vi "Set Matrix - file.vi"(5 "double array":dbl[][](array[numeric]), 6 "cmplx double array":cdb[][](array[numeric]), 7 "string array":string[](array[string]), 8 "error in (no error)":errorcluster, 10 "variable name":string, 11 "GOLPI ref. in":T1={"pipe handle"={"lv_proc.dll file path"=path "", "process instance handle"=[], "debug mode"=FALSE, "debug data"=[]}, "fast read timeout [ms]"=500, "fast read settle time [ms]"=10, "fast read to multiple [ms]"=1, "max elements per input line"=100, "slow read timeout [ms]"=5000, "stdin double format specifier"="%_16e", "max elements per stdout output column"=100, "console mode bitstream"=FALSE, "bitstream first read timeout [ms]"=1000, "bitstream read timeout [ms]"=50, "struct transfer possible"=FALSE}) -> (0 "error out":errorcluster, 3 "GOLPI ref. out":T1={"pipe handle"={"lv_proc.dll file path"=path "", "process instance handle"=[], "debug mode"=FALSE, "debug data"=[]}, "fast read timeout [ms]"=500, "fast read settle time [ms]"=10, "fast read to multiple [ms]"=1, "max elements per input line"=100, "slow read timeout [ms]"=5000, "stdin double format specifier"="%_16e", "max elements per stdout output column"=100, "console mode bitstream"=FALSE, "bitstream first read timeout [ms]"=1000, "bitstream read timeout [ms]"=50, "struct transfer possible"=FALSE})   [LabVIEW 2013, in "GOLPI library.lvlib"]
doc: "Saves LabVIEW variable into temporary file and loads it into GNU Octave. Supported are reals (doubles), complex and strings. Only one input can be nonempty array."
uses:
  GOLPI library.lvlib
  Public/GOLPI reference Type Def.ctl
  LV Process source distribution/Pipe Handle.ctl
  Type Definitions/Custom Error Codes Enum Type Def.vi
  LV Process source distribution/LV Process library.lvlib
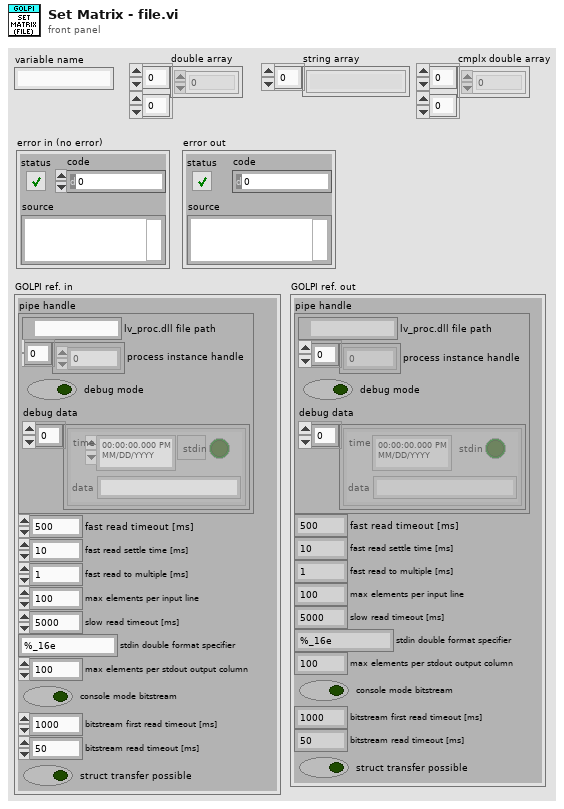
[diagram p1: front panel]
types:
  T1 = typedef "GOLPI library.lvlib/GOLPI reference Type Def.ctl" = cluster{"pipe handle":T2, "fast read timeout [ms]":u32, "fast read settle time [ms]":u32, "fast read to multiple [ms]":u32, "max elements per input line":u32, "slow read timeout [ms]":u32, "stdin double format specifier":string, "max elements per stdout output column":u32, "console mode bitstream":bool, "bitstream first read timeout [ms]":u32, "bitstream read timeout [ms]":u32, "struct transfer possible":bool}
  T2 = typedef "LV Process library.lvlib/Pipe Handle.ctl" = cluster{"lv_proc.dll file path":path, "process instance handle":u32[], "debug mode":bool, "debug data":cluster{"time":timestamp, "stdin":bool, "data":string}[]}
  T3 = typedef "GOLPI library.lvlib/Custom Error Codes Enum Type Def.vi" = enum16{"no error", "00 working directory PAR1 missing", "01 octave binary PAR1 missing", "02 octave report error PAR1", "03 empty output last cmd PAR1", "04 missing temporary file PAR1", "05 pwd PAR 1 not exist", "06 oct package not installed", "10 var PAR1 not string, vect", "11 var PAR1 not num, scal, ~compl", "12 var PAR1 not num, scal, compl", "13 var PAR1 not num, vect, ~compl", "14 var PAR1 not num, vect, compl", "15 var PAR1 not num, mat, ~compl", "16 var PAR1 not num, mat, ~compl", "30 read timeout", "60 bitstream transport failed", "61 bitstream decode error PAR1", "62 bitstream cannot be set", "70 struct transfer not possible", "80 struct: cluster elem. PAR1 not implem.", "81 struct: structure field PAR1 not implem.", "82 struct: size mismatch of PAR1", "83 struct: type mismatch of PAR1", "98 internal error", "99 not finished"}
  T4 = enum16{"open", "replace", "create", "open or create", "replace or create", "replace or create with confirmation"}
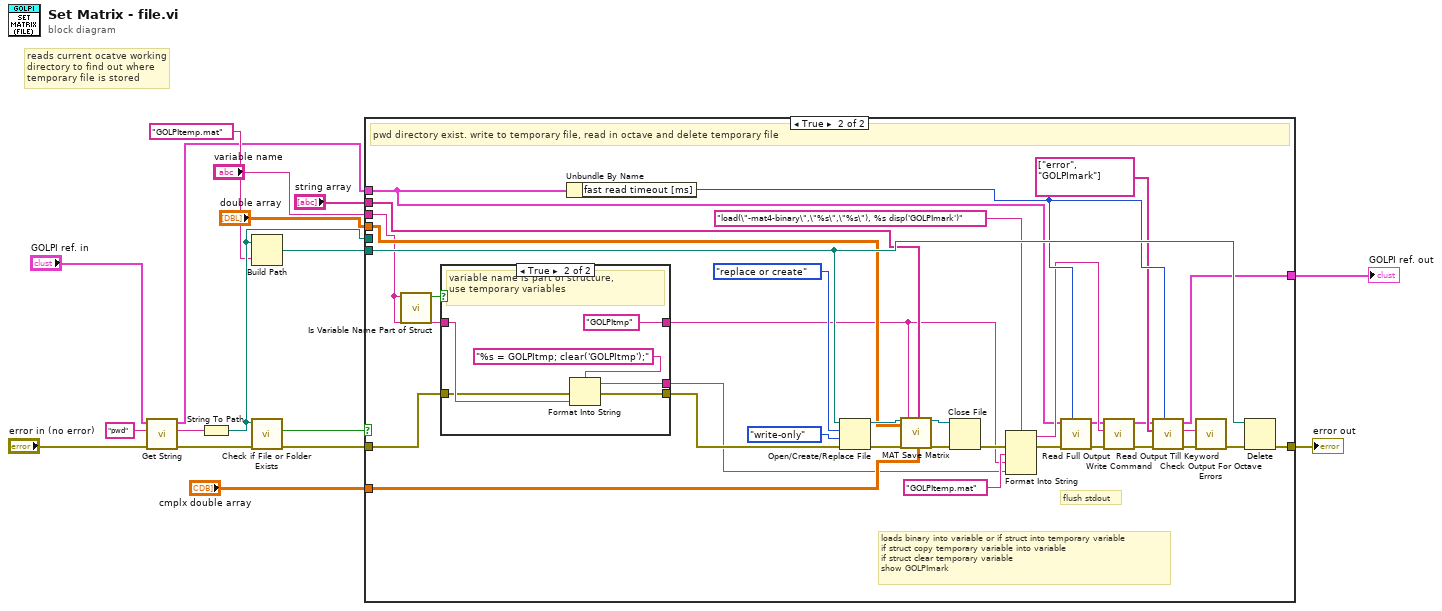
[diagram p0: block diagram]
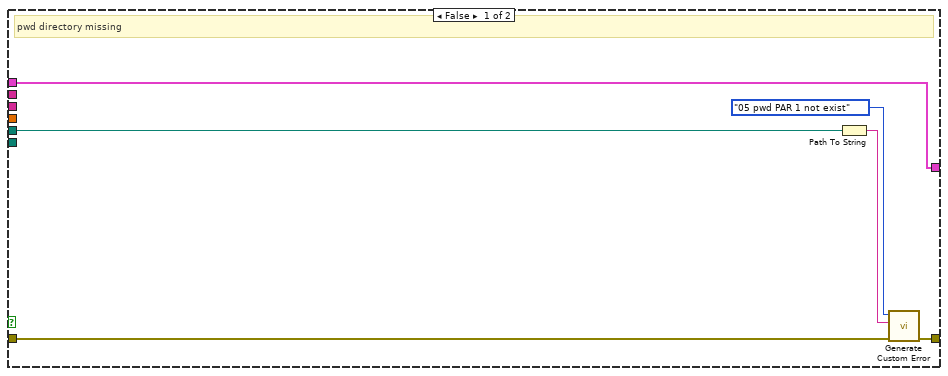
[diagram p2: hidden frame]
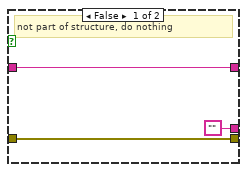
[diagram p3: hidden frame]
diagram:
  # "reads current ocatve working\ndirectory to find out where\ntemporary file is stored"
  n1 = call "Get String.vi"("error in"="error in (no error)", "variable name"="pwd", "GOLPI ref. in"="GOLPI ref. in") -> ("error out"=w7:errorcluster, "value"=w5:string, "GOLPI ref. out"=w1:T1)  [unwired: 6 in]
  n2 = String To Path(string=w5) -> (path=w3:path)
  n3 = Build Path(base path=w3, name or relative path="GOLPItemp.mat") -> (appended path=w4:path)
  n4 = call <vilib>:"Check if File or Folder Exists.vi"("error in (no error)"=w7, "path"=w3) -> ("error out"=w9:errorcluster, "file or folder exists?"=w8:bool)  [unwired: 7 in, 1 out]
  n5 = case shown="True" w8 {
    tunnel: [w22 w54] -> w17
    tunnel: w9 -> [w23 w27]
    tunnel: w4 -> [_ w53]
    tunnel: w3 -> [w19 _]
    tunnel: "variable name" -> [_ w28]
    tunnel: "string array" -> [_ w48]
    tunnel: "double array" -> [_ w47]
    tunnel: "cmplx double array" -> [_ w46]
    tunnel: w1 -> [w18 w31]
    tunnel: [w18 w30] -> w10
    frame False {
      # "pwd directory missing"
      n6 = Path To String(path=w19) -> (string=w20:string)
      n7 = call "Generate Custom Error.vi"("error in"=w23, "PAR1"=w20, "GOLPI error"=Custom_Error_Codes_Enum_Type_Def.vi."05 pwd PAR 1 not exist" ("Enum")) -> ("error out"=w22:errorcluster)  [unwired: 8 in]
    }
    frame True {
      # "loads binary into variable or if struct into temporary variable\nif struct copy temporary variable into variable\nif struct clear temporary variable\nshow GOLPImark"
      # "flush stdout"
      # "pwd directory exist. write to temporary file, read in octave and delete temporary file"
      n8 = call "Is Variable Name Part of Struct.vi"("variable name"=w28) -> ("Is part of struct?"=w29:bool)  [unwired: 10 in]
      n9 = case shown="True" w29 {
        tunnel: w28 -> [w59 w63]
        tunnel: [w59 "GOLPItmp" ("format string")] -> w24
        tunnel: w27 -> [w58 w62]
        tunnel: [w58 w61] -> w26
        tunnel: ["" w60] -> w25
        frame False {
          # "not part of structure, do nothing"
        }
        frame True {
          # "variable name is part of structure,\nuse temporary variables"
          n10 = Format Into String(format string="%s = GOLPItmp; clear('GOLPItmp');", error in=w62, w63) -> (resulting string=w60:string, error out=w61:errorcluster)  [unwired: 1 in]
        }
      }
      n11 = Unbundle By Name(w31) -> ("fast read timeout [ms]"=w45:u32)
      n12 = Open/Create/Replace File(file path (use dialog)=w53, error in=w26, operation (0:open)=T4."replace or create", access (0:read/write)=enum16{"read/write", "read-only", "write-only"}."write-only") -> (refnum out=w52:refnum<file>, error out=w51:errorcluster)  [unwired: 2 in, 1 out]
      n13 = call "MAT Save Matrix.vi"("Ref Num"=w52, "DBL"=w47, "error in"=w51, "Matrix Name"=w24, "STR"=w48, "CDB"=w46) -> ("Dup Ref Num"=w49:refnum<file>, "error out"=w50:errorcluster)  [unwired: 12 in]
      n14 = Close File(refnum=w49, error in=w50) -> (error out=w33:errorcluster)  [unwired: 1 out]
      n15 = Format Into String(format string="load(\"-mat4-binary\",\"%s\",\"%s\"), %s disp('GOLPImark')", error in=w33, "GOLPItemp.mat" ("name or relative path"), w24, w25) -> (resulting string=w42:string, error out=w36:errorcluster)  [unwired: 1 in]
      n16 = call "Read Full Output.vi"("timeout [ms]"=w45, "error in"=w36, "GOLPI ref. in"=w31) -> ("error out"=w35:errorcluster, "GOLPI ref. out"=w34:T1)  [unwired: 5 in, 2 out]
      n17 = call "Write Command.vi"("error in"=w35, "command"=w42, "GOLPI ref. in"=w34) -> ("error out"=w37:errorcluster, "GOLPI ref. out"=w40:T1)  [unwired: 7 in]
      n18 = call "Read Output Till Keyword.vi"("timeout [ms]"=w45, "error in"=w37, "keywords"=string[] ["error", "GOLPImark"], "GOLPI ref. in"=w40) -> ("error out"=w38:errorcluster, "read buffer"=w39:string, "GOLPI ref. out"=w30:T1)  [unwired: 4 in, 1 out]
      n19 = call "Check Output For Octave Errors.vi"("error in"=w38, "read buffer"=w39) -> ("error out"=w32:errorcluster)  [unwired: 9 in]
      n20 = Delete(path (use dialog)=w53, error in=w32) -> (error out=w54:errorcluster)  [unwired: 3 in, 2 out]
    }
  }
  "error out" <- w17
  "GOLPI ref. out" <- w10
